vi "mount_controls.vi"(9 "Mode":i32, 10 "Desired Position":dbl[](array[numeric]) format="%#_13g") -> (1 "Coupling":dbl format="%#_g%%")   [LabVIEW 2020]
uses:
  C:/Users/359167/Documents/LabVIEW_ws/Thorlabs.MotionControl.FTD2xx_Net.dll
  359167/Documents/LabVIEW_ws/Thorlabs.MotionControl.FTD2xx_Net.dll
  <vilib>/Utility/file.llb/Write Delimited Spreadsheet (DBL).vi
  <vilib>/Utility/file.llb/Read Delimited Spreadsheet (DBL).vi
panel:
  in  "# of channels":i32=4
  out "Channel and Absolute Pos.":dbl[][](array[numeric])
  in  "Path 3":path=path "C:/Users/359167/Documents/saved_position.csv"
  in  "Path 2":path=path "C:/Users/359167/Documents/saved_position.csv"
  in  "Path":path=path "C:/Users/359167/Documents/saved_position.csv"
  out "Device ID":string[](array[string])
  out "Serial #":string[](array[string])
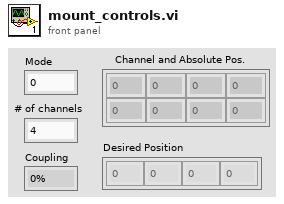
[diagram p1: front panel]
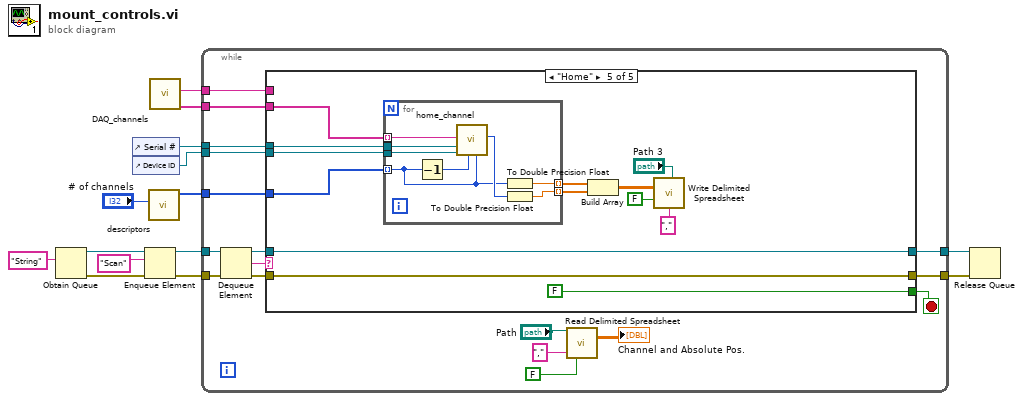
[diagram p0: block diagram]
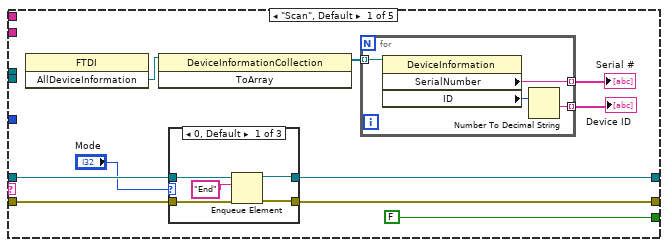
[diagram p2: hidden frame]
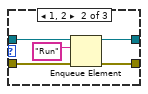
[diagram p3: hidden frame]
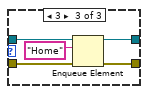
[diagram p4: hidden frame]
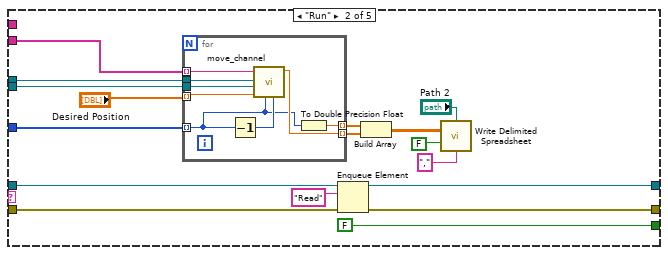
[diagram p5: hidden frame]
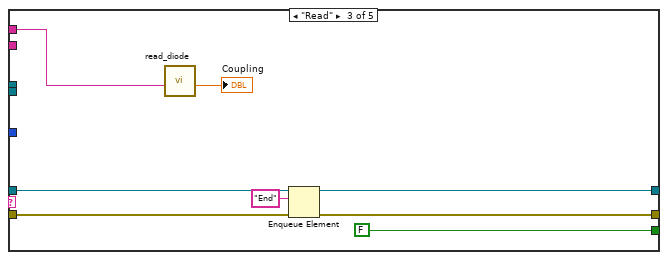
[diagram p6: hidden frame]
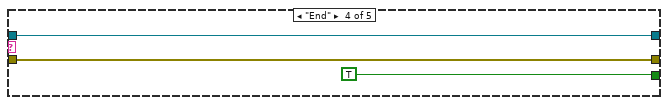
[diagram p7: hidden frame]
diagram:
  n1 = Obtain Queue(element data type="String") -> (queue out=w13:refnum<queue>, error out=w14:errorcluster)  [unwired: 4 in, 1 out]
  n2 = control-ref of="Serial #"() -> (w7:refnum<vi>)
  n3 = control-ref of="Device ID"() -> (w6:refnum<vi>)
  n4 = Enqueue Element(queue=w13, element="Scan", error in (no error)=w14) -> (queue out=w11:refnum<queue>, error out=w9:errorcluster)  [unwired: 1 in, 1 out]
  n5 = call "descriptors.vi"("# of channels"="# of channels") -> ("channel #s"=w8:i32[])  [unwired: 7 in, 3 out]
  n6 = call "DAQ_channels.vi"() -> ("subset of DAQ channels"=w5:tag[], "Channel 0"=w1:tag)  [unwired: 9 in, 1 out]
  n7 = while {
    tunnel: w11 -> [w31]
    tunnel: w9 -> [w30]
    tunnel: w8 -> [w29]
    tunnel: w7 -> [w28]
    tunnel: w6 -> [w27]
    tunnel: w5 -> [w26]
    tunnel: [w18] -> w4
    tunnel: [w17] -> w3
    tunnel: w1 -> [w15]
    stop <- w16 stop-if-true
    n8 = Dequeue Element(queue=w31, error in (no error)=w30) -> (queue out=w24:refnum<queue>, element=w23:string, error out=w25:errorcluster)  [unwired: 1 in, 1 out]
    n9 = case shown="\"Home\"" w23 {
      tunnel: w25 -> [w36 w65 w93 w95 w98]
      tunnel: w24 -> [w37 w66 w92 w96 w99]
      tunnel: w26 -> [_ w77 _ _ w109]
      tunnel: w29 -> [_ w69 _ _ w102]
      tunnel: w28 -> [_ w68 _ _ w100]
      tunnel: w27 -> [_ w67 _ _ w101]
      tunnel: [w34 w63 w90 w96 w99] -> w18
      tunnel: [w33 w62 w89 w95 w98] -> w17
      tunnel: [FALSE FALSE FALSE TRUE FALSE] -> w16
      tunnel: w15 -> [_ _ w87 _ _]
      frame "Scan", Default {
        n10 = invoke class="FTDI" method="AllDeviceInformation"() -> ("AllDeviceInformation"=w41:refnum<k24>)  [unwired: 3 in, 2 out]
        n11 = invoke class="DeviceInformationCollection" method="ToArray"(reference=w41) -> ("ToArray"=w40:refnum<k24>[])  [unwired: 2 in, 2 out]
        n12 = case shown="0, Default" "Mode" {
          tunnel: w37 -> [w46 w51 w56]
          tunnel: w36 -> [w45 w50 w55]
          tunnel: [w42 w48 w53] -> w34
          tunnel: [w43 w47 w52] -> w33
          frame 0, Default {
            n13 = Enqueue Element(queue=w46, element="End", error in (no error)=w45) -> (queue out=w42:refnum<queue>, error out=w43:errorcluster)  [unwired: 1 in, 1 out]
          }
          frame 1, 2 {
            n14 = Enqueue Element(queue=w51, element="Run", error in (no error)=w50) -> (queue out=w48:refnum<queue>, error out=w47:errorcluster)  [unwired: 1 in, 1 out]
          }
          frame 3 {
            n15 = Enqueue Element(queue=w56, element="Home", error in (no error)=w55) -> (queue out=w53:refnum<queue>, error out=w52:errorcluster)  [unwired: 1 in, 1 out]
          }
        }
        n16 = for {
          tunnel: w40 -> [w60] mode=indexing
          tunnel: [w59] -> w38 mode=indexing
          tunnel: [w57] -> w39 mode=indexing
          n17 = property class="DeviceInformation"(reference=w60) -> ("SerialNumber"=w59:string, "ID"=w58:u32)  [unwired: 1 in, 2 out]
          n18 = Number To Decimal String(number=w58) -> (decimal integer string=w57:string)  [unwired: 1 in]
        }
        "Serial #" <- w38
        "Device ID" <- w39
      }
      frame "Run" {
        n19 = for {
          tunnel: w77 -> [w81] mode=indexing
          tunnel: "Desired Position" -> [w80] mode=indexing
          tunnel: [w85] -> w72 mode=indexing
          tunnel: [w84] -> w71 mode=indexing
          tunnel: w69 -> [w78] mode=indexing
          tunnel: w68 -> [w82]
          tunnel: w67 -> [w83]
          n20 = Decrement(x=w78) -> (x-1=w79:i32)
          n21 = call "move_channel.vi"("file index"=w79, "Mount Channel"=w78, "Desired"=w80, "Device ID"=w83, "Serial #"=w82, "DAQ Channel"=w81) -> ("Absolute Position"=w85:dbl)  [unwired: 3 in, 2 out]
          n22 = To Double Precision Float(number=w78) -> (double precision float=w84:dbl)
        }
        n23 = Enqueue Element(queue=w66, element="Read", error in (no error)=w65) -> (queue out=w63:refnum<queue>, error out=w62:errorcluster)  [unwired: 1 in, 1 out]
        n24 = Build Array(w71, w72) -> (w70:dbl[][])
        n25 = call-poly <vilib>:"Write Delimited Spreadsheet.vi"("file path (dialog if empty)"="Path 2", "2D data"=w70, "append to file? (new file:F)"=FALSE, "delimiter (\\t)"="," ("delimiter (\\t)")) -> ()  [unwired: 10 in, 2 out]
      }
      frame "Read" {
        n26 = call "read_diode.vi"("DAQmx Physical Channel"=w87) -> ("% Coupled"=→"Coupling":dbl)  [unwired: 10 in]
        n27 = Enqueue Element(queue=w92, element="End", error in (no error)=w93) -> (queue out=w90:refnum<queue>, error out=w89:errorcluster)  [unwired: 1 in, 1 out]
      }
      frame "End" {
      }
      frame "Home" {
        n28 = for {
          tunnel: w109 -> [w117] mode=indexing
          tunnel: [w116] -> w104 mode=indexing
          tunnel: [w114] -> w103 mode=indexing
          tunnel: w102 -> [w112] mode=indexing
          tunnel: w101 -> [w111]
          tunnel: w100 -> [w110]
          n29 = Decrement(x=w112) -> (x-1=w113:i32)
          n30 = call "home_channel.vi"("Channel"=w112, "file index"=w113, "Device ID"=w111, "Serial #"=w110, "DAQ channel"=w117) -> ("Zero"=w115:i32)  [unwired: 5 in, 1 out]
          n31 = To Double Precision Float(number=w112) -> (double precision float=w116:dbl)
          n32 = To Double Precision Float(number=w115) -> (double precision float=w114:dbl)
        }
        n33 = Build Array(w104, w103) -> (w105:dbl[][])
        n34 = call-poly <vilib>:"Write Delimited Spreadsheet.vi"("file path (dialog if empty)"="Path 3", "2D data"=w105, "append to file? (new file:F)"=FALSE, "delimiter (\\t)"="," ("delimiter (\\t)")) -> ()  [unwired: 10 in, 2 out]
      }
    }
    n35 = call-poly <vilib>:"Read Delimited Spreadsheet.vi"("file path (dialog if empty)"="Path", "transpose? (F)"=FALSE, "delimiter (\\t)"="," ("delimiter (\\t)")) -> ("all rows"=→"Channel and Absolute Pos.":dbl[][])  [unwired: 7 in, 5 out]
  }
  n36 = Release Queue(queue=w4, error in (no error)=w3) -> ()  [unwired: 1 in, 3 out]
